vi "MoveAfterReference Core.vi"(8 "error in (no error)":errorcluster, 9 "Raw-Position":dbl, 10 "AxisNumber":u8, 11 "CS++Motor in":refnum<class "CS++Motor.lvclass">) -> (0 "error out":errorcluster, 3 "CS++Motor out":refnum<class "CS++Motor.lvclass">)   [LabVIEW 2015, in "CS++Motor.lvlib" / "CS++Motor.lvclass"]
doc: "Starts a movement to the reference switch of this axis. Once the motor reaches the reference switch it should slowly move down from the switch, resets the internal step counter and moves to the desired absolute position.\n\nThis function is a combination of <b>Move.vi</b> and <b>ReferenceMove.vi</b>."
uses:
  CS++Motor.lvclass
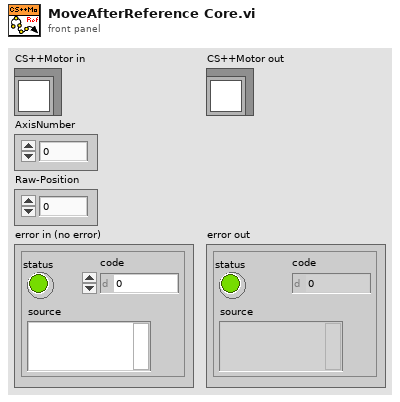
[diagram p1: front panel]
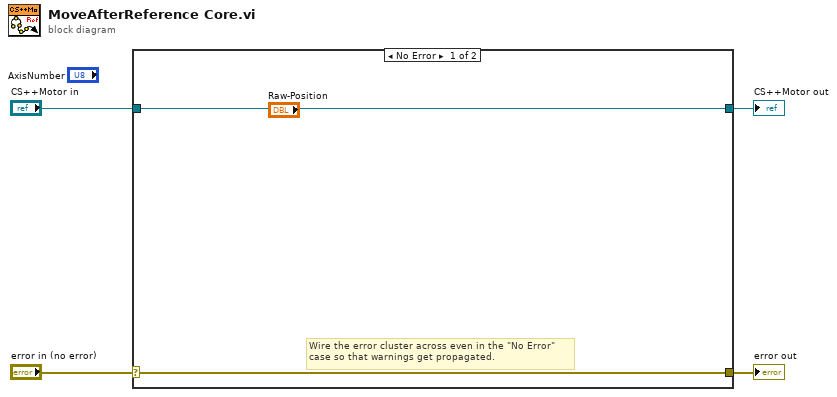
[diagram p0: block diagram]
diagram:
  n1 = case shown="No Error" "error in (no error)" {
    selector: "error in (no error)" -> [w5 w8]
    tunnel: [w5 w8] -> w3
    tunnel: [w6 w7] -> w1
    tunnel: "CS++Motor in" -> [w6 w7]
    frame No Error {
      # "Wire the error cluster across even in the \"No Error\"\ncase so that warnings get propagated."
    }
    frame Error {
    }
  }
  "error out" <- w3
  "CS++Motor out" <- w1
